vi "CPP Convert.vi"(8 "error in (no error)":errorcluster, 11 "configuration scripts":path) -> (0 "error out":errorcluster, 3 "I2C Commands":u16[][](array[numeric]))   [LabVIEW 2025, in "I2C Bus Monitor.lvclass"]
uses:
  I2C Bus Monitor.lvclass
  <vilib>/Utility/error.llb/Trim Whitespace One-Sided.vi
  I2C Bus Monitor.lvclass/I2C Bus Monitor.ctl
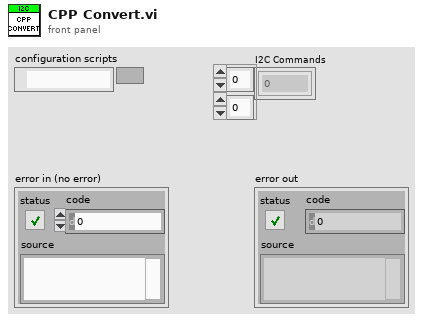
[diagram p1: front panel]
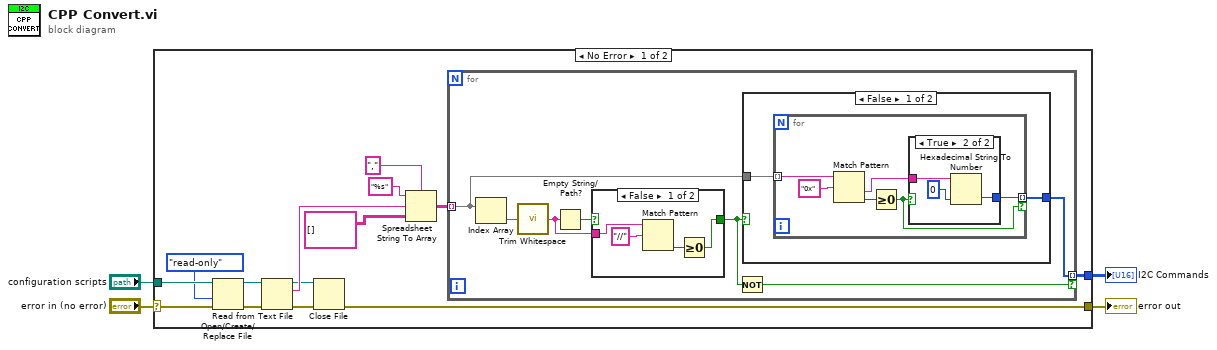
[diagram p0: block diagram]
diagram:
  n1 = case shown="No Error" "error in (no error)" {
    selector: "error in (no error)" -> [w16 w42]
    tunnel: [w18 w42] -> w4
    tunnel: "configuration scripts" -> [w17 _]
    tunnel: [w15 _] -> w1
    frame No Error {
      n2 = Open/Create/Replace File(file path (use dialog)=w17, error in=w16, access (0:read/write)=enum16{"read/write", "read-only", "write-only"}."read-only") -> (refnum out=w6:refnum<file>, error out=w7:errorcluster)  [unwired: 3 in, 1 out]
      n3 = Read from Text File(file (use dialog)=w6, error in=w7) -> (refnum out=w8:refnum<file>, text=w10:string, error out=w9:errorcluster)  [unwired: 2 in, 1 out]
      n4 = Close File(refnum=w8, error in=w9) -> (error out=w18:errorcluster)  [unwired: 1 out]
      n5 = Spreadsheet String To Array(delimiter (Tab)=",", format string="%s", spreadsheet string=w10, array type (2D Dbl)=string[][] []) -> (array=w14:string[][])
      n6 = for {
        tunnel: w14 -> [w19] mode=indexing
        tunnel: [w21] -> w15 mode=indexing if=w20
        n7 = Index Array(array=w19) -> (element=w25:string)  [unwired: 1 in]
        n8 = call <vilib>:"Trim Whitespace.vi"("string"=w25) -> ("trimmed string"=w23:string)  [unwired: 1 in]
        n9 = Empty String/Path?(string/path=w23) -> (empty?=w24:bool)
        n10 = case shown="False" w24 {
          selector: w24 -> [_ w41]
          tunnel: [w37 w41] -> w22
          tunnel: w23 -> [w40 _]
          frame False {
            n11 = Match Pattern(string=w40, regular expression="//") -> (offset past match=w38:i32)  [unwired: 1 in, 3 out]
            n12 = Greater Or Equal To 0?(x=w38) -> (x >= 0?=w37:bool)
          }
          frame True {
          }
        }
        n13 = Not(x=w22) -> (.not. x?=w20:bool)
        n14 = case shown="False" w22 {
          tunnel: w19 -> [w27 _]
          tunnel: [w26 _] -> w21
          frame False {
            n15 = for {
              tunnel: w27 -> [w32] mode=indexing
              tunnel: [w29] -> w26 mode=indexing if=w28
              n16 = Match Pattern(string=w32, regular expression="0x") -> (after substring=w30:string, offset past match=w31:i32)  [unwired: 1 in, 2 out]
              n17 = Greater Or Equal To 0?(x=w31) -> (x >= 0?=w28:bool)
              n18 = case shown="True" w28 {
                tunnel: w30 -> [_ w36]
                tunnel: [_ w34] -> w29
                frame False {
                }
                frame True {
                  n19 = Hexadecimal String To Number(string=w36, default (0uL)=u16 0) -> (number=w34:u16)  [unwired: 1 in, 1 out]
                }
              }
            }
          }
          frame True {
          }
        }
      }
    }
    frame Error {
    }
  }
  "error out" <- w4
  "I2C Commands" <- w1
